vi "dmm_configure_volts.vi"(4 "Session Name":string="SampleDMM") -> (0 "error out":errorcluster)   [LabVIEW 2011]
doc: "This VI gets the session that Session Name specifies and converts it into an IVI instrument handle\nbefore calling an IviDmm class driver method to configure the measurement."
uses:
  <vilib>/addons/TestStand/_SMUtility.llb/Session Manager - Get Instrument Session (32-bit).vi
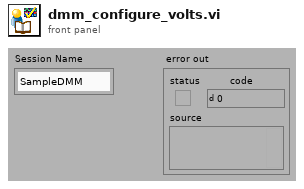
[diagram p1: front panel]
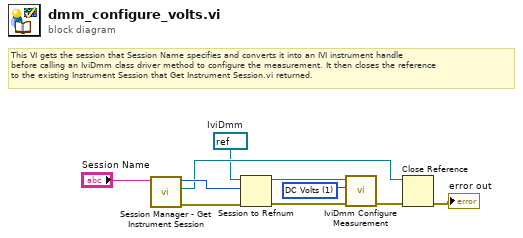
[diagram p0: block diagram]
diagram:
  w2 = refnum<k15> refnum  # IviDmm
  w6 = 1 items=["DC Volts"=1, "AC Volts"=2, "DC Current"=3, "AC Current"=4, "2 Wire Resistance"=5, "4 Wire Resistance"=101, "AC + DC Volts"=106, "AC + DC Current"=107, "Frequency"=104, "Period"=105, "Temperature"=108] ("measurement function (DC Volts)")
  # "This VI gets the session that Session Name specifies and converts it into an IVI instrument handle\nbefore calling an IviDmm class driver method to configure the measurement. It then closes the reference\nto the existing Instrument Session that Get Instrument Session.vi returned."
  n1 = call-poly <vilib>:"Session Manager - Get Instrument Session.vi"("Session Name"="Session Name") -> ("error out"=w9:errorcluster, "Instrument Session"=w4:refnum<k7>, "Driver Handle"=w10:u32)  [unwired: 8 in]
  n2 = Session to Refnum(4:w9, 6:w10, 7:w2) -> (0:w8:errorcluster, 3:w7:refnum<k15>)
  n3 = call <vilib>:"IviDmm Configure Measurement.vi"("error in (no error)"=w8, "measurement function (DC Volts)"=w6, "instrument handle"=w7) -> ("error out"=w5:errorcluster)  [unwired: 7 in, 1 out]
  n4 = Close Reference(reference=w4, error in (no error)=w5) -> (error out=→"error out":errorcluster)
